vi "Get Log Config.vi"(8 "error in (no error)":errorcluster) -> (0 "error out":errorcluster, 3 "Log Config":T1={"Log Level"=enum."WARNING"})   [LabVIEW 2020, in "RxnRover.lvlib" / "logging.lvlib"]
doc: "Gets the current logging configuration."
uses:
  logging.lvlib
  Log Levels.ctl
  Log Config.ctl
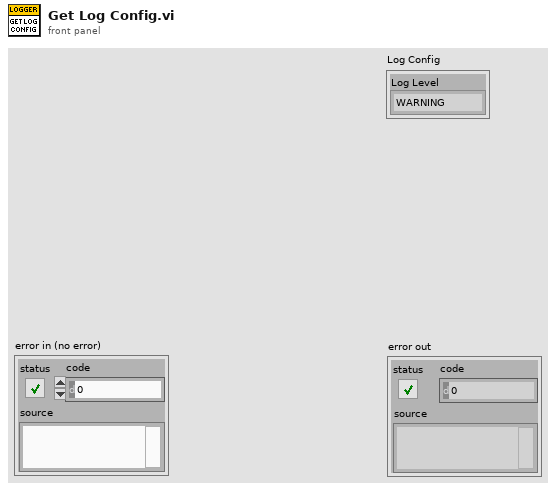
[diagram p1: front panel]
types:
  T1 = typedef "RxnRover.lvlib/logging.lvlib/Log Config.ctl" = cluster{"Log Level":T2}
  T2 = typedef "RxnRover.lvlib/logging.lvlib/Log Levels.ctl" = enum16{"NOTSET", "DEBUG", "INFO", "WARNING", "ERROR", "CRITICAL"}
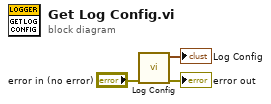
[diagram p0: block diagram]
diagram:
  n1 = call "Log Config.vi"("error in (no error)"="error in (no error)") -> ("error out"=→"error out":errorcluster, "Log Config out"=→"Log Config":T1)  [unwired: 9 in]
